vi "VSI Block Write Read Bytes.vi"(1 "IntervalTime":u32, 4 "BlockNum":u16, 5 "ReadBlockSize":u16, 6 "WriteBlockSize":u16, 7 "pWriteData":u8[](array[numeric])=array[10240 elements], 9 "SPIIndex":i32, 10 "DevIndex":i32, 11 "DevType":i32) -> (2 "function return":i32, 3 "pReadData":u8[](array[numeric]))   [LabVIEW 2010, in "ControlSPI.lvlib"]
doc: "int WINAPI VSI_BlockWriteReadBytes(int DevType,int DevIndex,int SPIIndex,unsigned char *pWriteData,unsigned short WriteBlockSize,unsigned char *pReadData,unsigned short ReadBlockSize,unsigned short BlockNum,unsigned int IntervalTime);"
uses:
  ControlSPI.lvlib
  ControlSPI/Ginkgo_Driver.dll
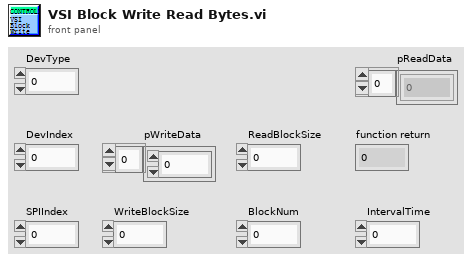
[diagram p1: front panel]
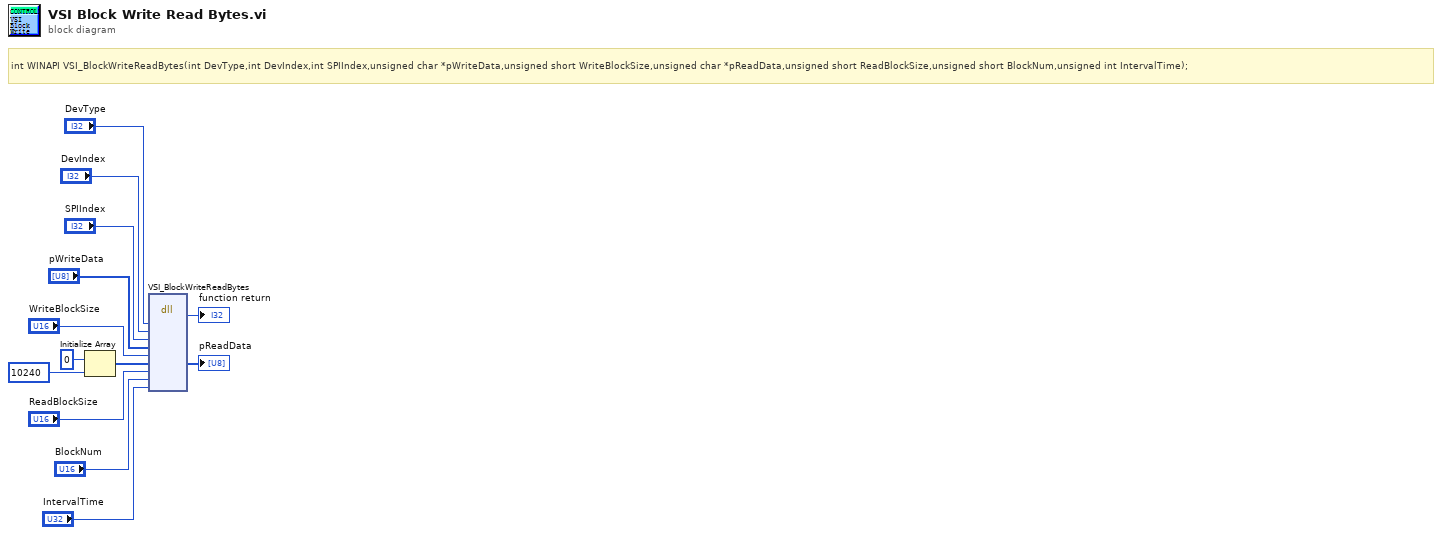
[diagram p0: block diagram]
diagram:
  # "int WINAPI VSI_BlockWriteReadBytes(int DevType,int DevIndex,int SPIIndex,unsigned char *pWriteData,unsigned short WriteBlockSize,unsigned char *pReadData,unsigned short ReadBlockSize,unsigned short BlockNum,unsigned int IntervalTime);"
  n1 = Initialize Array(u8 0 ("element"), 10240 ("dimension size")) -> (w7:u8[])
  n2 = dll-call lib="E:/Project/vt_ginkgo/truck/Ginkgo Driver/vs2010/Ginkgo_USB-I2C&SPI&CAN_API_v2.0.3.3/lib/labview_32bit/ControlSPI/Ginkgo_Driver.*" fn="VSI_BlockWriteReadBytes"("DevType"="DevType", "DevIndex"="DevIndex", "SPIIndex"="SPIIndex", "pWriteData"="pWriteData", "WriteBlockSize"="WriteBlockSize", "pReadData"=w7, "ReadBlockSize"="ReadBlockSize", "BlockNum"="BlockNum", "IntervalTime"="IntervalTime") -> (→"function return":i32, "pReadData"=→"pReadData":u8[])  [unwired: 11 in, 2 out]
